vi "Find Event Structure Timeout Constant.vi"(8 "error in (no error)":errorcluster, 11 "EventStructure in":refnum<vi>) -> (0 "error out":errorcluster, 2 "DigitalNumericConstant out":refnum<vi>)   [LabVIEW 2020, in "JKI State Machine API.lvlib" / "JKI SM.lvclass"]
uses:
  JKI SM.lvclass
  JKI SM.lvclass/JKI SM.ctl
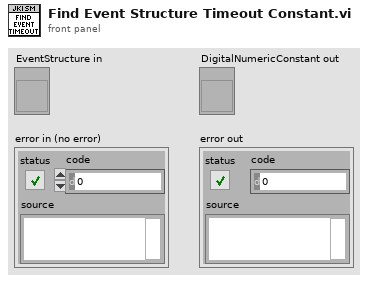
[diagram p1: front panel]
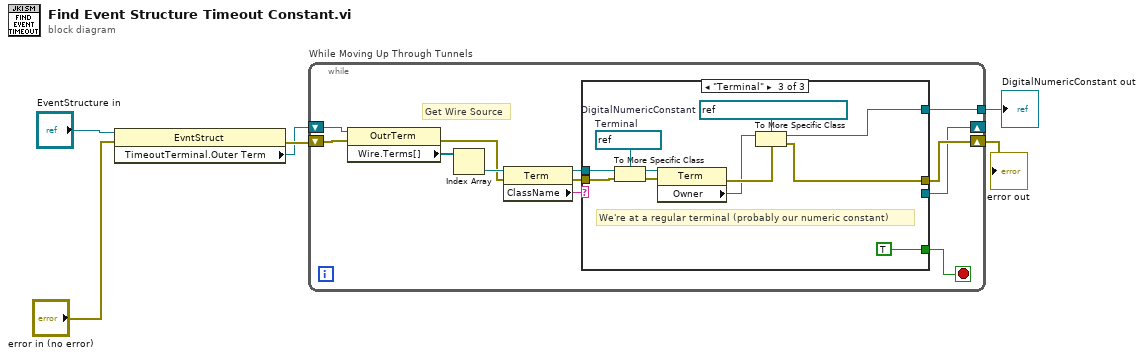
[diagram p0: block diagram]
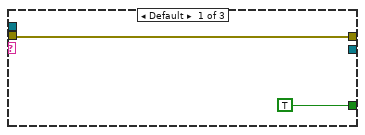
[diagram p2: hidden frame]
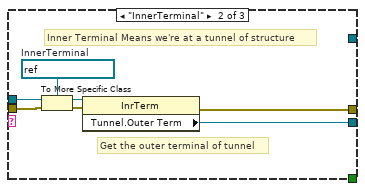
[diagram p3: hidden frame]
diagram:
  n1 = property class="EvntStruct"(reference="EventStructure in", error in="error in (no error)") -> (error out=w6:errorcluster, "TimeoutTerminal.Outer Term"=w3:refnum<vi>)  [unwired: 1 out]
  n2 = while "While Moving Up Through Tunnels" {
    shift-right: [w11] -> w5
    shift-left: w6 -> [w17]
    shift-right: [w10] -> _
    shift-left: w3 -> [w9]
    tunnel: [w7] -> w4
    stop <- w8 stop-if-true
    # "Get Wire Source"
    n3 = property class="OutrTerm"(reference=w9, error in=w17) -> (error out=w13:errorcluster, "Wire.Terms[]"=w18:refnum<vi>[])  [unwired: 1 out]
    n4 = Index Array(array=w18) -> (element=w16:refnum<vi>)  [unwired: 1 in]
    n5 = property class="Term"(reference=w16, error in=w13) -> (reference out=w14:refnum<vi>, error out=w12:errorcluster, "ClassName"=w15:string)
    n6 = case shown="\"Terminal\"" w15 {
      tunnel: w14 -> [_ w27 w38]
      tunnel: w12 -> [w20 w24 w35]
      tunnel: [w20 w22 w33] -> w11
      tunnel: [_ w21 _] -> w10
      tunnel: [TRUE _ TRUE] -> w8
      tunnel: [_ _ w31] -> w7
      frame Default {
      }
      frame "InnerTerminal" {
        w25 = refnum<vi> refnum  # InnerTerminal
        # "Get the outer terminal of tunnel"
        # "Inner Terminal Means we're at a tunnel of structure"
        n7 = To More Specific Class(target class=w25, reference=w27, error in=w24) -> (specific class reference=w26:refnum<vi>, error out=w23:errorcluster)
        n8 = property class="InrTerm"(reference=w26, error in=w23) -> (error out=w22:errorcluster, "Tunnel.Outer Term"=w21:refnum<vi>)  [unwired: 1 out]
      }
      frame "Terminal" {
        w32 = refnum<vi> refnum  # DigitalNumericConstant
        w36 = refnum<vi> refnum  # Terminal
        # "We're at a regular terminal (probably our numeric constant)"
        n9 = To More Specific Class(target class=w36, reference=w38, error in=w35) -> (specific class reference=w37:refnum<vi>, error out=w34:errorcluster)
        n10 = property class="Term"(reference=w37, error in=w34) -> (error out=w30:errorcluster, "Owner"=w28:refnum<vi>)  [unwired: 1 out]
        n11 = To More Specific Class(target class=w32, reference=w28, error in=w30) -> (specific class reference=w31:refnum<vi>, error out=w33:errorcluster)
      }
    }
  }
  "error out" <- w5
  "DigitalNumericConstant out" <- w4
